vi "Get Sparse Marker Indexes [SM] Core.vi"(8 "error in (no error)":errorcluster, 9 "Marker Name (\"\")":string caption="marker name (\"\")", 10 "Indexes Array Size":i64 caption="indexes array size" format="%.0g", 11 "CS++Fgen in":refnum<class "CS++Fgen.lvclass">) -> (0 "error out":errorcluster, 1 "Indexes Array":i64[](array[numeric]) caption="indexes array", 2 "Indexes Actual Size":i64 caption="indexes actual size", 3 "CS++Fgen out":refnum<class "CS++Fgen.lvclass">)   [LabVIEW 2013, in "CS++Fgen.lvlib" / "CS++Fgen.lvclass"]
doc: "The VI returns the coerced indexes associated with the sparse marker. You can use the following VIs to specify indexes:\n\n- IviFgen Configure Sparse Marker [SM] VI\n- IviFgen Set Sparse Marker Indexes [SM] VI\n\nNote:\n\n(1) This VI is part of the IviFgenSparseMarker [SM] extension group."
uses:
  CS++Fgen.lvclass
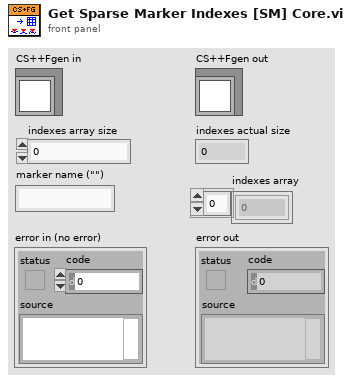
[diagram p1: front panel]
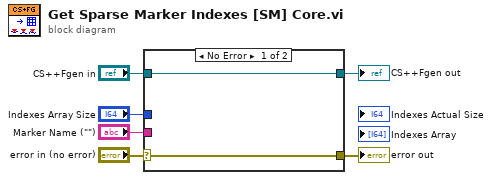
[diagram p0: block diagram]
diagram:
  n1 = case shown="No Error" "error in (no error)" {
    selector: "error in (no error)" -> [w7 w10]
    tunnel: [w7 w10] -> w5
    tunnel: [w8 w9] -> w3
    tunnel: "CS++Fgen in" -> [w8 w9]
    tunnel: "Marker Name (\"\")" -> [_ _]
    tunnel: "Indexes Array Size" -> [_ _]
    frame No Error {
    }
    frame Error {
    }
  }
  "error out" <- w5
  "CS++Fgen out" <- w3
